vi "Tab Navigate (SubVI).vi"(0 "Active CtlRef":refnum<vi>, 7 "Active Refs":T1) -> ()   [LabVIEW 2010]
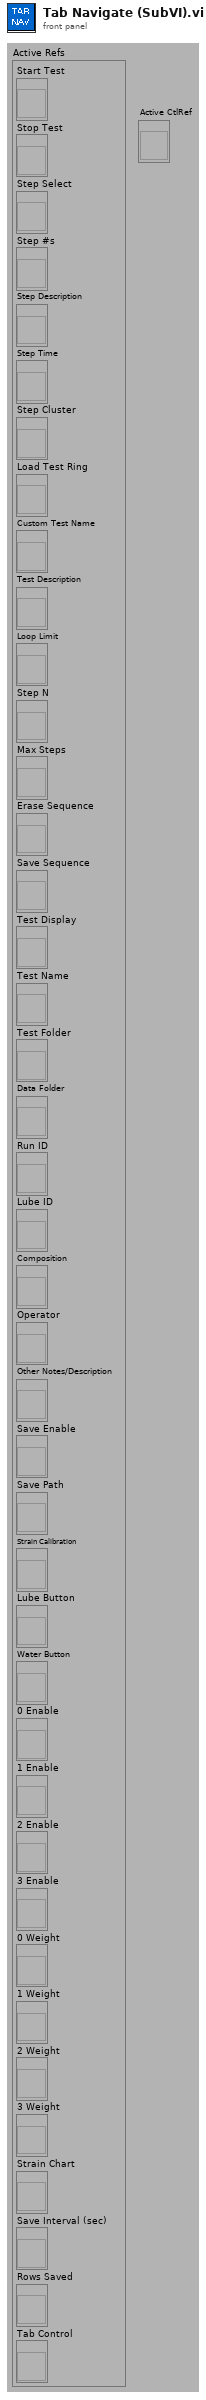
[diagram p1: front panel]
types:
  T1 = cluster{"Start Test":refnum<vi>, "Stop Test":refnum<vi>, "Step Select":refnum<vi>, "Step #s":refnum<vi>, "Step Description":refnum<vi>, "Step Time":refnum<vi>, "Step Cluster":refnum<vi>, "Load Test Ring":refnum<vi>, "Custom Test Name":refnum<vi>, "Test Description":refnum<vi>, "Loop Limit":refnum<vi>, "Step N":refnum<vi>, "Max Steps":refnum<vi>, "Erase Sequence":refnum<vi>, "Save Sequence":refnum<vi>, "Test Display":refnum<vi>, "Test Name":refnum<vi>, "Test Folder":refnum<vi>, "Data Folder":refnum<vi>, "Run ID":refnum<vi>, "Lube ID":refnum<vi>, "Composition":refnum<vi>, "Operator":refnum<vi>, "Other Notes/Description":refnum<vi>, "Save Enable":refnum<vi>, "Save Path":refnum<vi>, "Strain Calibration":refnum<vi>, "Lube Button":refnum<vi>, "Water Button":refnum<vi>, "0 Enable":refnum<vi>, "1 Enable":refnum<vi>, "2 Enable":refnum<vi>, "3 Enable":refnum<vi>, "0 Weight":refnum<vi>, "1 Weight":refnum<vi>, "2 Weight":refnum<vi>, "3 Weight":refnum<vi>, "Strain Chart":refnum<vi>, "Save Interval (sec)":refnum<vi>, "Rows Saved":refnum<vi>, "Tab Control":refnum<vi>}
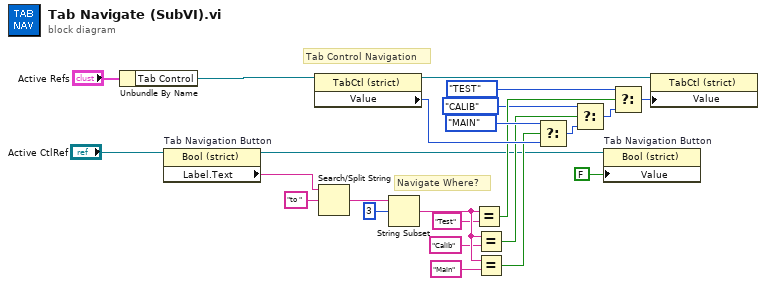
[diagram p0: block diagram]
diagram:
  # "Tab Control Navigation"
  # "Navigate Where?"
  n1 = Unbundle By Name("Active Refs") -> ("Tab Control"=w4:refnum<vi>)
  n2 = property on="Tab Navigation Button" class="Bool (strict)"(reference="Active CtlRef") -> (reference out=w1:refnum<vi>, "Label.Text"=w3:string)  [unwired: 1 in, 1 out]
  n3 = property class="TabCtl (strict)"(reference=w4) -> (reference out=w22:refnum<vi>, "Value"=w21:enum32{"MAIN", "CALIB", "TEST"})  [unwired: 1 in, 1 out]
  n4 = Search/Split String(string=w3, search string/char (-)="to ") -> (match + rest of string=w6:string)  [unwired: 1 in, 2 out]
  n5 = String Subset(string=w6, offset (0)=3 ("y")) -> (substring=w15:string)  [unwired: 1 in]
  n6 = Equal?(x=w15, y="Test") -> (x = y?=w13:bool)
  n7 = Equal?(x=w15, y="Calib") -> (x = y?=w12:bool)
  n8 = Equal?(x=w15, y="Main") -> (x = y?=w17:bool)
  n9 = Select(t=enum32{"MAIN", "CALIB", "TEST"}."MAIN" ("Value"), s=w17, f=w21) -> (s? t:f=w19:enum32{"MAIN", "CALIB", "TEST"})
  n10 = Select(t=enum32{"MAIN", "CALIB", "TEST"}."CALIB" ("Value"), s=w12, f=w19) -> (s? t:f=w16:enum32{"MAIN", "CALIB", "TEST"})
  n11 = property on="Tab Navigation Button" class="Bool (strict)"(reference=w1, "Value"=FALSE) -> ()  [unwired: 1 in, 2 out]
  n12 = Select(t=enum32{"MAIN", "CALIB", "TEST"}."TEST" ("Value"), s=w13, f=w16) -> (s? t:f=w20:enum32{"MAIN", "CALIB", "TEST"})
  n13 = property class="TabCtl (strict)"(reference=w22, "Value"=w20) -> ()  [unwired: 1 in, 2 out]
